vi "mlink_dio_set_dir.vi"(8 "error in (no error)":errorcluster, 9 "direction":T2, 10 "bank":T1=1 items=["DIO1...8"=1, "DIO9...16"=2, "DIO17...24"=3, "DIO25...32"=4], 11 "connection ID":i32=-1) -> (0 "error out":errorcluster, 3 "connection ID out":i32)   [LabVIEW 2009, in "MicroDAQ.lvlib" / "mlink.lvlib"]
doc: "This function sets DIO bank direction. The DIO bank contains eight DIO channels (bank 1 -DIO1...8, bank 2 - DIO9....16, bank 3 - DIO17...24, bank 4 - DIO25...32). The function allows DIO bank direction change if it is supported by MicroDAQ hardware."
uses:
  <instrlib>/MicroDAQ/Mlink library wraper/mlink.lvlib
  <instrlib>/MicroDAQ/Tools/DIO set direction argument.ctl
  <instrlib>/MicroDAQ/Tools/Digital IO channels.ctl
  <instrlib>/MicroDAQ/MLink32.dll
  <instrlib>/MicroDAQ/MicroDAQ.lvlib
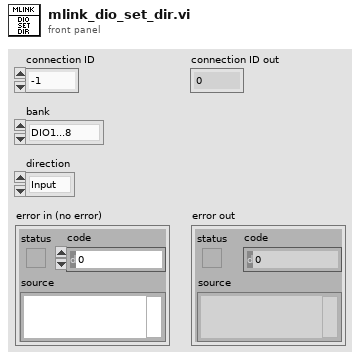
[diagram p1: front panel]
types:
  T1 = typedef "MicroDAQ.lvlib/Digital IO channels.ctl" = u8
  T2 = typedef "MicroDAQ.lvlib/DIO set direction argument.ctl" = enum8{"Input", "Output"}
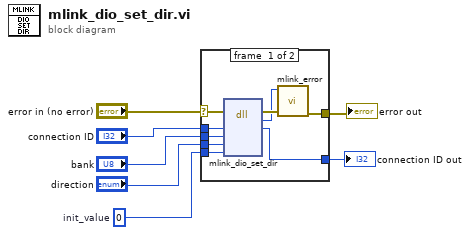
[diagram p0: block diagram]
diagram:
  w4 = u8 0  # init_value
  n1 = case shown="No Error" "error in (no error)" {
    selector: "error in (no error)" -> [w14 w18]
    tunnel: "connection ID" -> [w16 w17]
    tunnel: [w15 w17] -> w6
    tunnel: w4 -> [w13 _]
    tunnel: [w11 w18] -> w3
    tunnel: "bank" -> [w9 _]
    tunnel: "direction" -> [w8 _]
    frame #0 {
      n2 = dll-call lib="C:/Program Files (x86)/National Instruments/LabVIEW 2009/instr.lib/MicroDAQ/MLink32.dll" fn="mlink_dio_set_dir"(error in=w14, "connection ID"=w16, "pin"=w9, "dir"=w8, "init_value"=w13) -> (error out=w12:errorcluster, "return type"=w10:i32, "connection ID"=w15:i32)  [unwired: 5 in, 1 out]
      n3 = call <instrlib>:"mlink_error.vi"("error in (no error)"=w12, "error code"=w10) -> ("error out"=w11:errorcluster)  [unwired: 9 in]
    }
    frame #1 {
    }
  }
  "connection ID out" <- w6
  "error out" <- w3
